vi "CheckPressureStabilityForDecay.vi"(8 "error in":errorcluster, 11 "S1 in":refnum<class "S2.lvclass">) -> (0 "error out":errorcluster, 3 "S1 out":refnum<class "S2.lvclass">)   [LabVIEW 2018]
uses:
  S2.lvclass
  Public Controls/ReportHeader.ctl
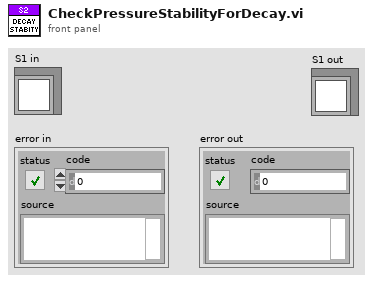
[diagram p1: front panel]
types:
  T1 = typedef "S2.lvclass/ReportHeader.ctl" = string
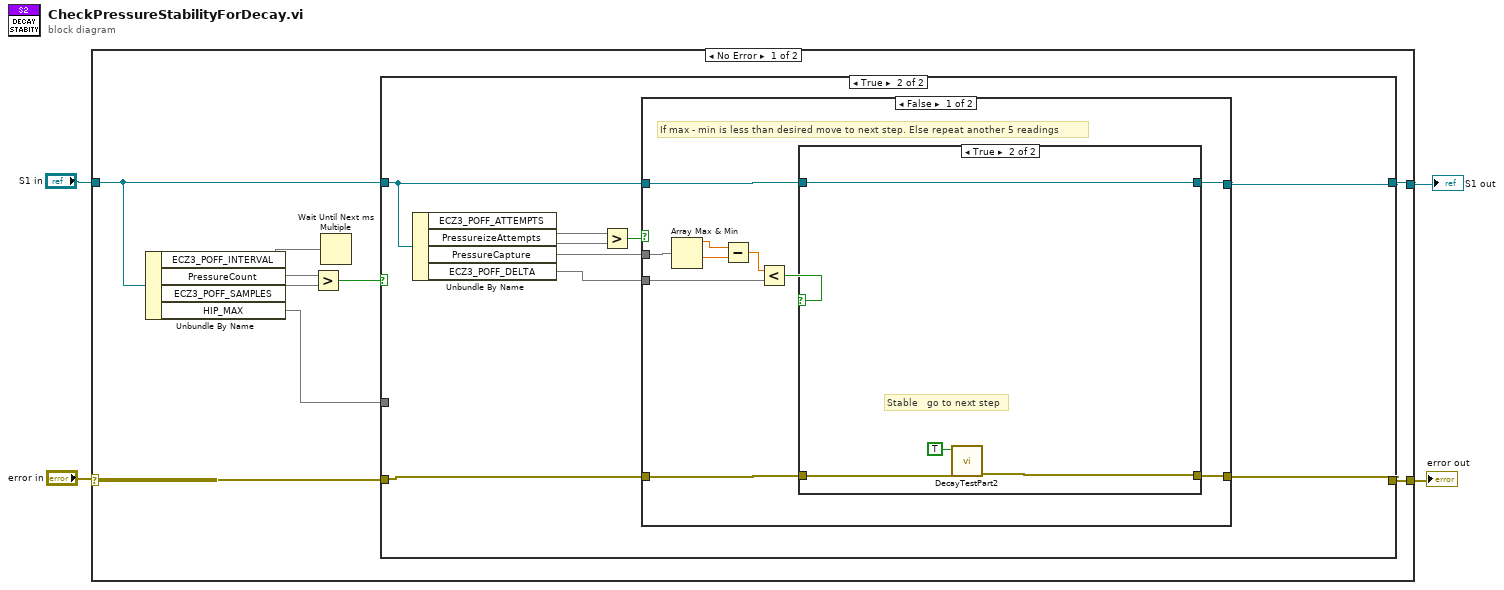
[diagram p0: block diagram]
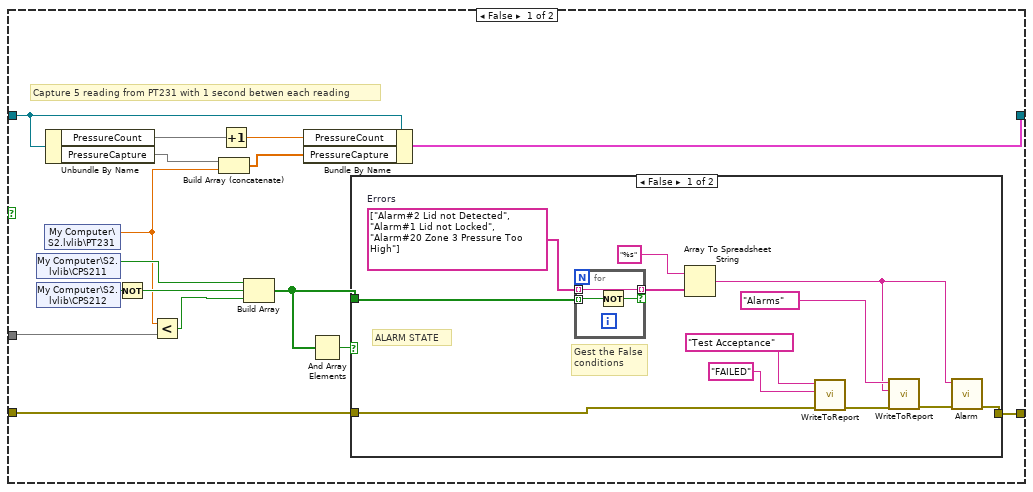
[diagram p2: hidden frame]
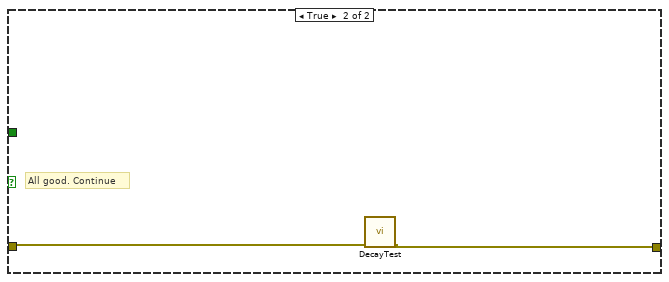
[diagram p3: hidden frame]
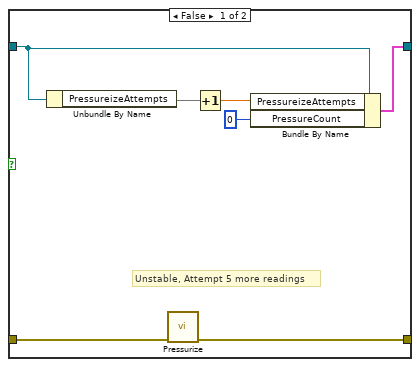
[diagram p4: hidden frame]
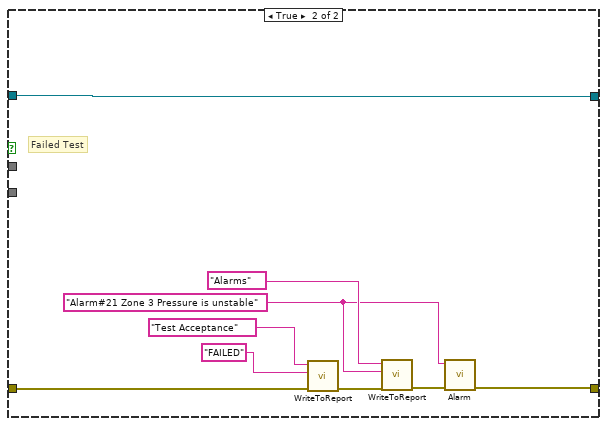
[diagram p5: hidden frame]
diagram:
  n1 = case shown="No Error" "error in" {
    selector: "error in" -> [w13 w87]
    tunnel: [w11 w87] -> w4
    tunnel: "S1 in" -> [w10 w86]
    tunnel: [w12 w86] -> w1
    frame No Error {
      n2 = Unbundle By Name(w10) -> ("ECZ3_POFF_INTERVAL"=w6, "PressureCount"=w7, "ECZ3_POFF_SAMPLES"=w8, "HIP_MAX"=w5)
      n3 = Greater?(x=w7, y=w8) -> (0:w9:bool)
      n4 = Wait Until Next ms Multiple(millisecond multiple=w6) -> ()  [unwired: 1 out]
      n5 = case shown="True" w9 {
        tunnel: [w29 w55] -> w11
        tunnel: w13 -> [w23 w54]
        tunnel: w10 -> [w22 w50]
        tunnel: [w21 w49] -> w12
        tunnel: w5 -> [w17 _]
        frame False {
          # "Capture 5 reading from PT231 with 1 second betwen each reading"
          n6 = shared-variable "My Computer\\S2.lvlib\\CPS211"() -> (w25:bool)  [unwired: 1 in, 1 out]
          n7 = shared-variable "My Computer\\S2.lvlib\\CPS212"() -> (w24:bool)  [unwired: 1 in, 1 out]
          n8 = shared-variable "My Computer\\S2.lvlib\\PT231"() -> (w15:dbl)  [unwired: 1 in, 1 out]
          n9 = Unbundle By Name(w22) -> ("PressureCount"=w19, "PressureCapture"=w16)
          n10 = Not(x=w24) -> (.not. x?=w18:bool)
          n11 = Less?(x=w15, y=w17) -> (x < y?=w28:bool)
          n12 = Build Array (concatenate)(w16, w15) -> (w14:dbl[])
          n13 = Increment(x=w19) -> (x+1=w20:dbl)
          n14 = Build Array(w25, w18, w28) -> (w26:bool[])
          n15 = Bundle By Name(cluster=w22, "PressureCount"=w20, "PressureCapture"=w14) -> (w21:cluster{})
          n16 = And Array Elements(Boolean array=w26) -> (logical AND=w27:bool)
          n17 = case shown="False" w27 {
            tunnel: w23 -> [w36 w46]
            tunnel: [w38 w45] -> w29
            tunnel: w26 -> [w35 _]
            frame False {
              w34 = string[] ["Alarm#2 Lid not Detected", "Alarm#1 Lid not Locked", "Alarm#20 Zone 3 Pressure Too High"]  # Errors
              # "ALARM STATE"
              # "Gest the False\nconditions"
              n18 = for {
                tunnel: w35 -> [w43] mode=indexing
                tunnel: w34 -> [w44] mode=indexing
                tunnel: [w44] -> w33 mode=indexing if=w42
                n19 = Not(x=w43) -> (.not. x?=w42:bool)
              }
              n20 = Array To Spreadsheet String(array=w33, 3:"%s" ("format string")) -> (spreadsheet string=w31:string)  [unwired: 1 in]
              n21 = call "WriteToReport.vi"("error in"=w36, "Value"="FAILED", "Header"=T1 "Test Acceptance") -> ("error out"=w41:errorcluster)  [unwired: 8 in]
              n22 = call "WriteToReport.vi"("error in"=w41, "Value"=w31, "Header"="Alarms") -> ("error out"=w39:errorcluster)  [unwired: 8 in]
              n23 = call "Alarm.vi"("error in"=w39, "Alarm"=w31) -> ("error out"=w38:errorcluster)  [unwired: 9 in]
            }
            frame True {
              # "All good. Continue"
              n24 = call "DecayTest.vi"("error in"=w46) -> ("error out"=w45:errorcluster)  [unwired: 10 in]
            }
          }
        }
        frame True {
          n25 = Unbundle By Name(w50) -> ("ECZ3_POFF_ATTEMPTS"=w47, "PressureizeAttempts"=w52, "PressureCapture"=w53, "ECZ3_POFF_DELTA"=w48)
          n26 = Greater?(x=w52, y=w47) -> (0:w51:bool)
          n27 = case shown="False" w51 {
            tunnel: [w57 w83] -> w55
            tunnel: w54 -> [w60 w81]
            tunnel: w53 -> [w65 _]
            tunnel: w50 -> [w59 w78]
            tunnel: [w58 w78] -> w49
            tunnel: w48 -> [w56 _]
            frame False {
              # "If max - min is less than desired move to next step. Else repeat another 5 readings"
              n28 = Array Max & Min(array=w65) -> (max value=w64:dbl, min value=w63:dbl)  [unwired: 2 out]
              n29 = Subtract(x=w64, y=w63) -> (x-y=w62:dbl)
              n30 = Less?(x=w62, y=w56) -> (x < y?=w61:bool)
              n31 = case shown="True" w61 {
                tunnel: w60 -> [w67 w76]
                tunnel: w59 -> [w71 w74]
                tunnel: [w72 w74] -> w58
                tunnel: [w66 w75] -> w57
                frame False {
                  # "Unstable, Attempt 5 more readings"
                  n32 = Unbundle By Name(w71) -> ("PressureizeAttempts"=w70)
                  n33 = call "Pressurize.vi"("error in"=w67) -> ("error out"=w66:errorcluster)  [unwired: 10 in]
                  n34 = Increment(x=w70) -> (x+1=w69:dbl)
                  n35 = Bundle By Name(cluster=w71, "PressureizeAttempts"=w69, "PressureCount"=u8 0) -> (w72:cluster{})
                }
                frame True {
                  # "Stable   go to next step"
                  n36 = call "DecayTestPart2.vi"("error in"=w76, "FirstCall(F)"=TRUE) -> ("error out"=w75:errorcluster)  [unwired: 9 in]
                }
              }
            }
            frame True {
              w77 = "Alarm#21 Zone 3 Pressure is unstable" ("String")
              # "Failed Test"
              n37 = call "WriteToReport.vi"("error in"=w81, "Value"="FAILED", "Header"=T1 "Test Acceptance") -> ("error out"=w85:errorcluster)  [unwired: 8 in]
              n38 = call "WriteToReport.vi"("error in"=w85, "Value"=w77, "Header"=T1 "Alarms") -> ("error out"=w84:errorcluster)  [unwired: 8 in]
              n39 = call "Alarm.vi"("error in"=w84, "Alarm"=w77) -> ("error out"=w83:errorcluster)  [unwired: 9 in]
            }
          }
        }
      }
    }
    frame Error {
    }
  }
  "error out" <- w4
  "S1 out" <- w1
